vi "GetAlazar_SaveToFile - ATS-SDK.vi"(1 "File Array":string[](array[string]), 2 "lines per plane":i32, 5 "Digitizer Settings":T8={"Digitizer delay (us) "=0.0, "rf points per line"=2048, "lines per plane"=128, "Samp Rate (Hz)"=100000000.0, "Additional dig delay (us)"=0.0, "Voltage Scale"=0.4, "Pre-Looks"=0, "Offset delay (us)"=0.0, "bits A/D"=8, "Avg Num"=1, "DigTimeOut"=5.0, "Rel Dig Delay"=0.0, "Dig Ch"=0, "LeCroyCluster"={"LeCroy Channels"=[TRUE, FALSE, FALSE, FALSE], "LC read pt offset"=0.0, "Sweep Avg"=FALSE}, "Main Digitizer"=enum."NI Digitizer", "Dig Config"=enum."Single channel", "Digitizer ID Cluster"={"Acqiris/Alazar/SP ID"=[], "NI Instr Handles"=[], "LeCroy VISA"="", "GaGe Handle"={"Handle"=0, "Sample size"=0, "Resolution"=0, "Offset"=0, "Channels"=0, "Boards"=0}, "ATS Ref"="ATS9350", "Acqiris Address"=["PCI::INSTR0"], "ADQRef"=refnum, "adq_cu_ptr"=refnum}, "Trigger Settings"={"Trig Source"=1, "Trig Coupling"=0, "Trig Slope"=0, "Level (mV)"=1500.0}, "Bulk Acq"=FALSE, "Bulk Start Indexes"=[], "Data Ref RF"=refnum, "NI ID/Channel"=[], "Total Dig CH"=1, "Xtra Ann Trig delay (us)"=10.0, "Fix Z Delay?"=FALSE, "One Way Transmission?"=FALSE, "Data Ref Log"=refnum} {"Trigger Settings"."Trig Slope" items=["Positive", "Negative"]; "Trigger Settings"."Level (mV)" format="%.2f"; "Trigger Settings"."Trig Coupling" items=["DC 1 MOhm", "AC 1 MOhm", "DC 50 Ohm", "AC 50 Ohm"]; "Trigger Settings"."Trig Source" items=["Chan 1", "External"]; "Rel Dig Delay" format="%.2f"; "DigTimeOut" format="%.2f"; "Avg Num" min=1; "Offset delay (us)" format="%.2f"; "Additional dig delay (us)" format="%.2f"; "Digitizer delay (us)" format="%.2f"}, 7 "Ann Array Params":T1={"Synth Foc?"=FALSE, "Focal Zones"=41, "Switch T/R"=0, "Trans Geometry (mm)"={"Transducer"=0, "Geo Focus"=12.0, "a (radius)"=3.0, "# of rings"=5, "kerf space "=0.1, "Center Freq"=12.0}, "Sub Ap Excite?"=FALSE, "Full Array Scan?"=FALSE, "Xmt/Rcv"={"XMIT"=[TRUE, TRUE, TRUE, TRUE, TRUE], "RCV"=[TRUE, TRUE, TRUE, TRUE, TRUE]}, "PulseSpacing (us)"=0.0, "Xmit Ring"=0, "XMIT CHS"=0, "RCV CHS"=0, "GPU?"=FALSE, "Save TIFF?"=FALSE, "downfactor"=1, "RCV 1CH"=0} {"RCV 1CH" items=["All", "1", "2", "3", "4", "5"]; "Trans Geometry (mm)"."Transducer" items=["6D 12R 40 MHz"=0, "10D 31R 20 MHz"=1, "10D 23R 20 MHz"=2, "6D 23R 40 MHz"=3, "4.5D 10.7R 40 MHz"=4, "9D 23.5R 20 MHz"=5, "9D 25.8R 20MHz"=6, "Enter"=99]; "Switch T/R" min=1 max=5 step=1}, 9 "AlazarCluster":T12, 11 "errorin":errorcluster, 12 "Motion Settings":T4={"No Motion?"=FALSE, "Motion System"=enum."NI 735x", "Motion Bd ID"=1, "Motion Profile"="SMAC1", "# Axis"=1, "Reverse Z axis?"=TRUE, "SMAC Axis"=0, "scan pair"=enum."y-(x) scan", "RT fps"=6.0, "Steps per mm"=[1000, 1000, 1000, 1000], "Motor Parameters"={"velocity ct/s"=[10000.0, 10000.0, 10000.0, 50000.0], "accel ct/s^2"=[50000.0, 50000.0, 50000.0, 200000.0]}, "One Way Scan"=FALSE, "Reverse One Way Scan"=FALSE, "Global Position (mm)"=[], "Plane"=0, "Distance between\nscan lines (um)"=0.0, "Distance between\nscan planes (um)"=0.0, "number of scan planes"=1, "Total steps in line"=0, "Xtra plane\ndistance  (um)"=100, "Xtra planes "=1, "Add Axis"=FALSE, "overshoot cts"=200, "BKPT Shift"=0, "Scan Start Time (ms)"=0, "ESP VISA"="GPIB::1::INSTR", "3rd Axis"=1, "GL Ref Out"=refnum, "Galil Address"=""} {"3rd Axis" items=["x", "y", "z", "w"]; "Xtra planes" min=1; "Xtra plane\ndistance  (um)" min=0; "Distance between\nscan planes (um)" format="%.2f"; "Distance between\nscan lines (um)" format="%.2f"; "SMAC Axis" items=["None"=0, "Axis 1"=1, "Axis 2"=2, "Axis 3"=3, "Axis 4"=4, "Axis 5"=5, "Axis 6"=6, "Axis 7"=7, "Axis 8"=8, "Vector Space 1"=17, "Vector Space 2"=18, "Vector Space 3"=19, "Vector Space 4"=20]; "Motion Bd ID" min=1 max=32 step=1}, 13 "Reverse?":bool) -> (3 "Gain Array":T14(array[cluster]), 6 "VGain (dB)":dbl, 14 "Raw VGain (scale)":dbl, 15 "error out":errorcluster)   [LabVIEW 2022 SP3]
uses:
  -DigitizerRoutines/DigitizerSettings.ctl
  -DigitizerRoutines/Digitizer.ctl
  -DigitizerRoutines/DigConfig.ctl
  -DigitizerRoutines/DigitizerID.ctl
  C:/Windows/System32/ADQAPI_dotNet_helper.dll
  Motion Controllers/NI_controller/-NI_MotionRoutines/MotionParameters.ctl
  Motion Controllers/NI_controller/-NI_MotionRoutines/MotionSys.ctl
  Motion Controllers/-MotionRoutines/ScanAxis.ctl
  Motion Controllers/-MotionRoutines/3rdAxis.ctl
  Annular Array/-AnnularRoutines/AnnularArray.ctl
  Annular Array/-AnnularRoutines/TransGeometry.ctl
  Annular Array/-AnnularRoutines/ArrayGeometry.ctl
  -ScanSystem/DataHandling/ReverseData.vi
panel:
  out "Voltage Scale":T13
  # "1-D and 2-D B scan settings"
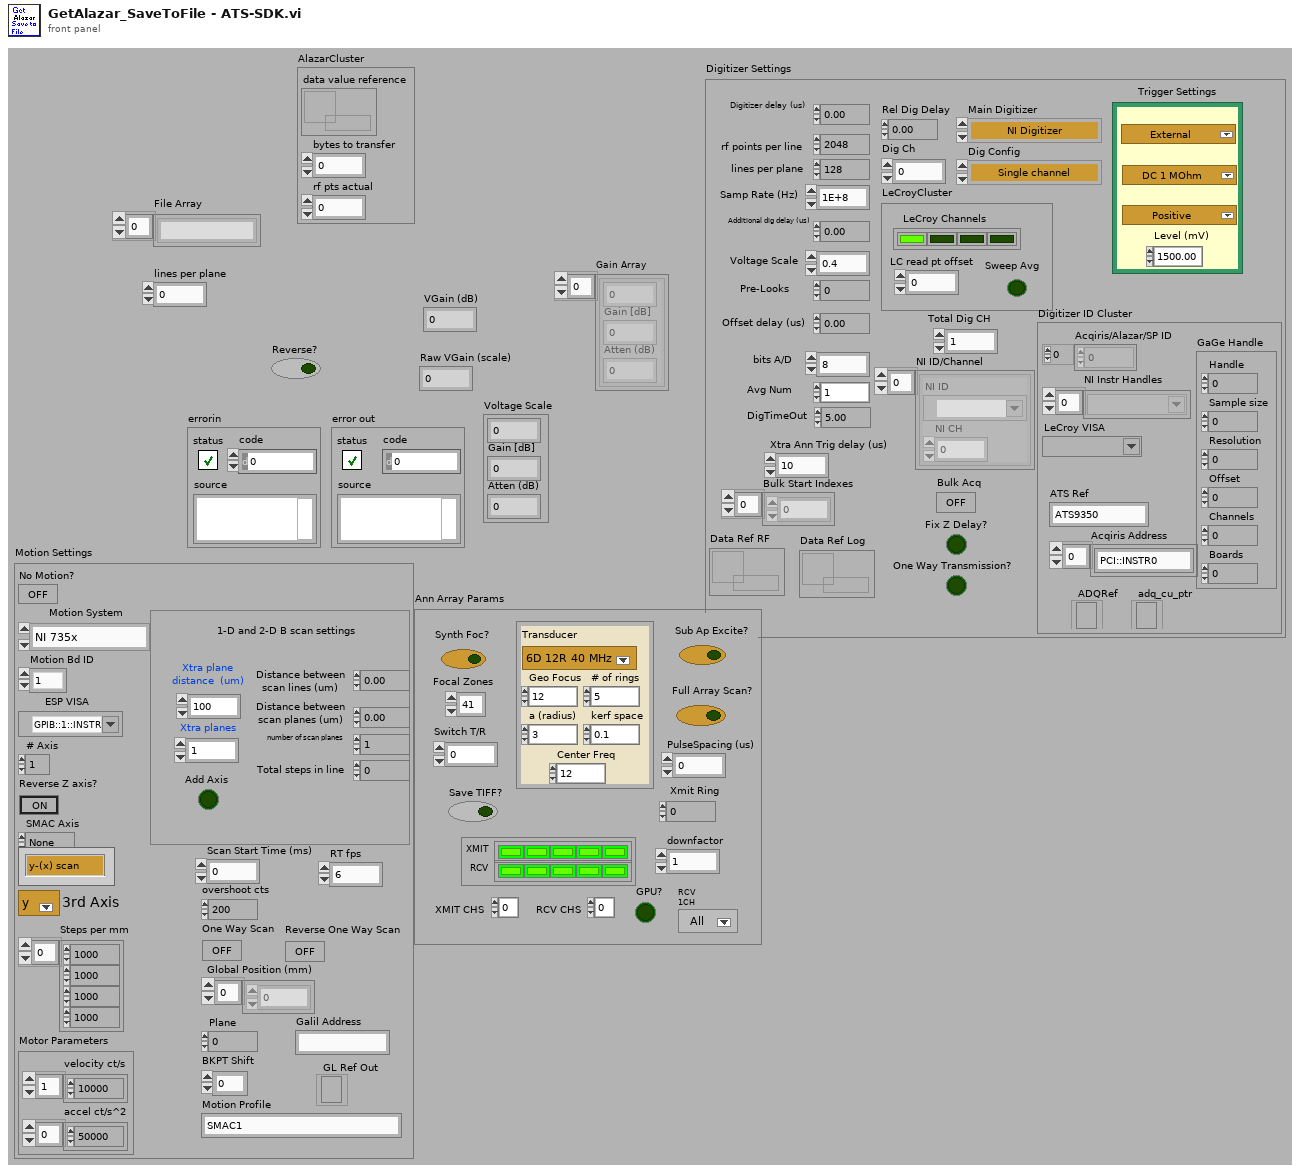
[diagram p1: front panel]
types:
  T1 = typedef "AnnularArray.ctl" = cluster{"Synth Foc?":bool, "Focal Zones":i16, "Switch T/R":i16, "Trans Geometry (mm)":T2, "Sub Ap Excite?":bool, "Full Array Scan?":bool, "Xmt/Rcv":cluster{"XMIT":bool[], "RCV":bool[]}, "PulseSpacing (us)":sgl, "Xmit Ring":i32, "XMIT CHS":u8, "RCV CHS":u8, "GPU?":bool, "Save TIFF?":bool, "downfactor":i32, "RCV 1CH":u16}
  T2 = typedef "TransGeometry.ctl" = cluster{"Transducer":T3, "Geo Focus":dbl, "a (radius)":dbl, "# of rings":i32, "kerf space ":dbl, "Center Freq":dbl}
  T3 = typedef "ArrayGeometry.ctl" = u16
  T4 = typedef "MotionParameters.ctl" = cluster{"No Motion?":bool, "Motion System":T5, "Motion Bd ID":u8, "Motion Profile":string, "# Axis":i8, "Reverse Z axis?":bool, "SMAC Axis":u16, "scan pair":T6, "RT fps":sgl, "Steps per mm":i32[], "Motor Parameters":cluster{"velocity ct/s":dbl[], "accel ct/s^2":dbl[]}, "One Way Scan":bool, "Reverse One Way Scan":bool, "Global Position (mm)":dbl[], "Plane":i32, "Distance between\nscan lines (um)":sgl, "Distance between\nscan planes (um)":sgl, "number of scan planes":i32, "Total steps in line":i32, "Xtra plane\ndistance  (um)":i32, "Xtra planes ":i32, "Add Axis":bool, "overshoot cts":i32, "BKPT Shift":i32, "Scan Start Time (ms)":u32, "ESP VISA":refnum<visa-resource-name>, "3rd Axis":T7, "GL Ref Out":refnum<k7>, "Galil Address":string}
  T5 = typedef "MotionSys.ctl" = enum16{"MM3000", "NI 735x", "Newport ESP", "No Motion Card", "Galil"}
  T6 = typedef "ScanAxis.ctl" = enum16{"y-(x) scan", "x-(y) scan", "z-(x) scan", "z-(y) scan", "y-(z) scan", "x-(z) scan", "w-(x) scan", "w-(y) scan", "w-(z) scan", "x-(w) scan", "y-(w) scan", "z-(w) scan"}
  T7 = typedef "3rdAxis.ctl" = u16
  T8 = typedef "DigitizerSettings.ctl" = cluster{"Digitizer delay (us) ":dbl, "rf points per line":i32, "lines per plane":i32, "Samp Rate (Hz)":dbl, "Additional dig delay (us)":dbl, "Voltage Scale":dbl, "Pre-Looks":i32, "Offset delay (us)":dbl, "bits A/D":i8, "Avg Num":i32, "DigTimeOut":sgl, "Rel Dig Delay":sgl, "Dig Ch":i32, "LeCroyCluster":cluster{"LeCroy Channels":bool[], "LC read pt offset":dbl, "Sweep Avg":bool}, "Main Digitizer":T9, "Dig Config":T10, "Digitizer ID Cluster":T11, "Trigger Settings":cluster{"Trig Source":u16, "Trig Coupling":u16, "Trig Slope":u16, "Level (mV)":dbl}, "Bulk Acq":bool, "Bulk Start Indexes":i32[], "Data Ref RF":refnum<data-value>, "NI ID/Channel":cluster{"NI ID":refnum<k15>, "NI CH":i32}[], "Total Dig CH":i32, "Xtra Ann Trig delay (us)":dbl, "Fix Z Delay?":bool, "One Way Transmission?":bool, "Data Ref Log":refnum<data-value>}
  T9 = typedef "Digitizer.ctl" = enum16{"Acqiris Digitizer", "NI Digitizer", "LeCroy", "GaGe", "AlazarTech", "No Digitizer", "Teledyne"}
  T10 = typedef "DigConfig.ctl" = enum16{"Single channel", "2 Chans w/ 2 Acqiris", "2 Chans w/ 1 Acqiris", "5-CH Pulser New", "5-CH pulser w/ ann array", "5-pass style ann array", "Empty"}
  T11 = typedef "DigitizerID.ctl" = cluster{"Acqiris/Alazar/SP ID":u32[], "NI Instr Handles":refnum<k15>[], "LeCroy VISA":refnum<visa-resource-name>, "GaGe Handle":cluster{"Handle":u32, "Sample size":u32, "Resolution":i32, "Offset":i32, "Channels":u32, "Boards":u32}, "ATS Ref":string, "Acqiris Address":string[], "ADQRef":refnum<k24>, "adq_cu_ptr":refnum<k24>}
  T12 = cluster{"data value reference":refnum<data-value>, "bytes to transfer":u32, "rf pts actual":u32}
  T13 = cluster{sgl, "Gain [dB]  ":sgl, "Atten (dB)":sgl}
  T14 = cluster{sgl, "Gain [dB]  ":sgl, "Atten (dB)":sgl}[]
  T15 = enum16{"big-endian, network order", "native, host order", "little-endian"}
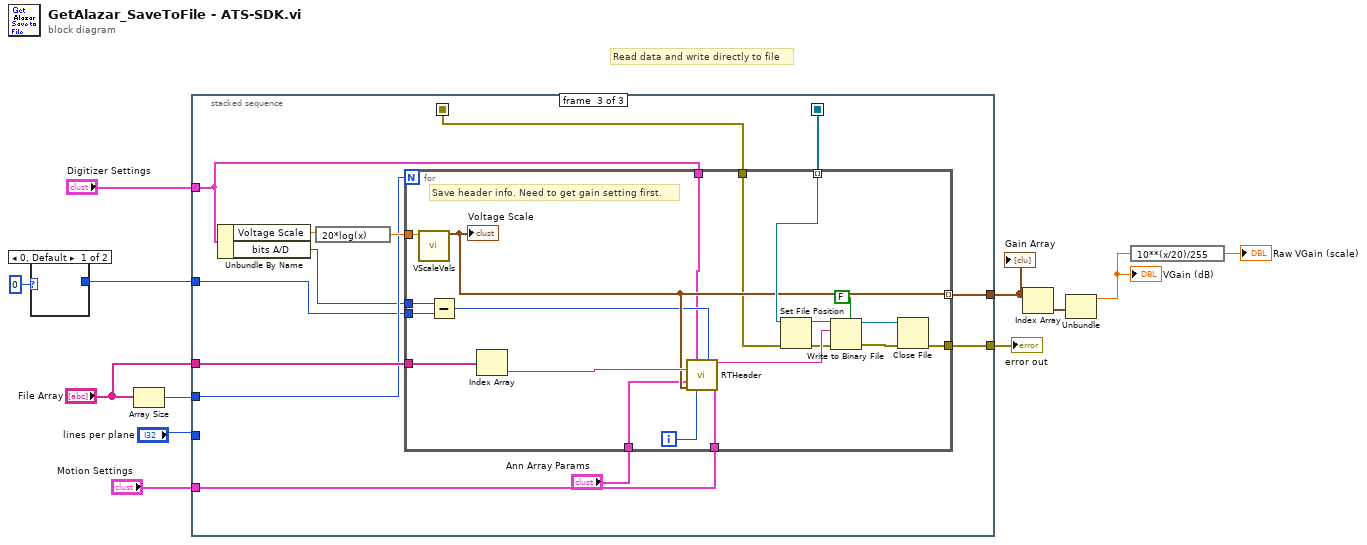
[diagram p0: block diagram]
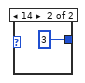
[diagram p2: hidden frame]
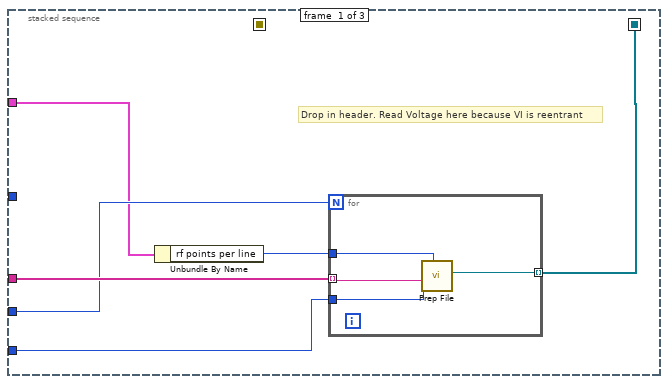
[diagram p3: hidden frame]
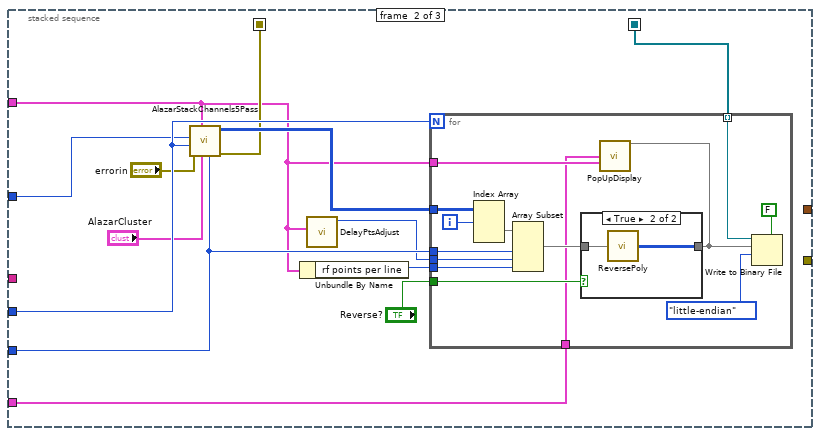
[diagram p4: hidden frame]
diagram:
  # "Read data and write directly to file"
  n1 = case shown="0, Default" i8 0 ("bits A/D") {
    tunnel: [_ u16 3 ("Extra Shift")] -> w5
    frame 0, Default {
    }
    frame 14 {
    }
  }
  n2 = Array Size(array="File Array") -> (size(s)=w9:i32)
  n3 = stacked-sequence {
    seq-local: [w19 _ _] -> [_ w34 w61]
    seq-local: [_ w29 _] -> [_ _ w57]
    tunnel: [_ _ w66] -> w2
    tunnel: "lines per plane" -> [w17 w35 _]
    tunnel: "File Array" -> [w18 _ w65]
    tunnel: w9 -> [w16 w33 w62]
    tunnel: [_ _ w63] -> w6
    tunnel: w5 -> [_ w31 w60]
    tunnel: "Digitizer Settings" -> [w15 w25 w56]
    tunnel: "Motion Settings" -> [_ w32 w58]
    frame #0 {
      # "Drop in header. Read Voltage here because VI is reentrant"
      n4 = Unbundle By Name(w15) -> ("rf points per line"=w14:i32)
      n5 = for {
        N: w16 -> [_]
        tunnel: [w23] -> w19 mode=indexing
        tunnel: w18 -> [w20] mode=indexing
        tunnel: w14 -> [w22]
        tunnel: w17 -> [w21]
        n6 = call "Prep File.vi"("Num Samps"=w22, "Num Segs"=w21, "File Name"=w20) -> ("refnum out"=w23:refnum<file>)  [unwired: 4 in, 1 out]
      }
    }
    frame #1 {
      n7 = call "AlazarStackChannels5Pass.vi"("lines per plane"=w35, "AlazarCluster"="AlazarCluster", "Digitizer Settings"=w25, "error in"="errorin", "Channels"=w33, "Extra Shift"=w31) -> ("error out"=w29:errorcluster, "ChStackDataOut"=w36:i16[][][])  [unwired: 2 in, 2 out]
      n8 = Unbundle By Name(w25) -> ("rf points per line"=w28:i32)
      n9 = call "DelayPtsAdjust.vi"("Digitizer Settings"=w25) -> ("PostDelayCorrection"=w24:u32)  [unwired: 9 in, 1 out]
      n10 = for {
        N: w33 -> [_]
        tunnel: w36 -> [w50]
        tunnel: w28 -> [w49]
        tunnel: w35 -> [w48]
        tunnel: "Reverse?" -> [w47]
        tunnel: w34 -> [w43] mode=indexing
        tunnel: w25 -> [w39]
        tunnel: w32 -> [w38]
        tunnel: w24 -> [w37]
        i -> [w41]
        n11 = Index Array(array=w50, index (dim 0)=w41) -> (element=w42:i16[][])  [unwired: 2 in]
        n12 = Array Subset(array=w42, length (row)=w48, index (col)=w37, length (col)=w49) -> (w46:i16[][])  [unwired: 1 in]
        n13 = case shown="True" w47 {
          tunnel: [w51 w53] -> w40
          tunnel: w46 -> [w51 w52]
          frame False {
          }
          frame True {
            n14 = call-poly "ReversePoly.vi"("Array in"=w52) -> ("Array out"=w53:i16[][])
          }
        }
        n15 = call "PopUpDisplay.vi"("Data"=w40, "Motion Settings In"=w38, "Digitizer Settings"=w39) -> ()  [unwired: 13 in]
        n16 = Write to Binary File(file (use dialog)=w43, data=w40, 5:FALSE ("prepend array or string size? (T)"), 9:T15."little-endian" ("byte order (0:big-endian, network order)")) -> ()  [unwired: 2 in, 3 out]
      }
    }
    frame #2 {
      n17 = Unbundle By Name(w56) -> ("Voltage Scale"=w55:dbl, "bits A/D"=w54:i8)
      n18 = expression code="20*log(x)"(w55) -> (w64:dbl)
      n19 = for {
        N: w62 -> [_]
        tunnel: [w86] -> w66
        tunnel: w65 -> [w85]
        tunnel: [w75] -> w63 mode=indexing
        tunnel: w64 -> [w77]
        tunnel: w61 -> [w76] mode=indexing
        tunnel: w60 -> [w74]
        tunnel: w56 -> [w72]
        tunnel: w58 -> [w71]
        tunnel: "Ann Array Params" -> [w69]
        tunnel: w57 -> [w68]
        tunnel: w54 -> [w67]
        i -> [w70]
        # "Save header info. Need to get gain setting first."
        n20 = call "VScaleVals.vi"("Full Scale"=w77) -> ("Voltage Scale"=w75:T13)  [unwired: 8 in, 2 out]
        "Voltage Scale" <- w75
        n21 = Subtract(x=w67, y=w74) -> (x-y=w73:u16)
        n22 = Index Array(array=w85) -> (element=w78:string)  [unwired: 1 in]
        n23 = call "RTHeader.vi"("Digitizer Settings"=w72, "Dig Word Size"=w73, "File Name In"=w78, "Ann Array Params"=w69, "Votage scaling"=w75, "Pulser Channel"=w70, "Motion Settings"=w71) -> ("Header String Out"=w81:string)  [unwired: 7 in, 1 out]
        n24 = Set File Position(refnum=w76, error in=w68) -> (refnum out=w80:refnum<file>, error out=w79:errorcluster)  [unwired: 2 in]
        n25 = Write to Binary File(file (use dialog)=w80, data=w81, error in=w79, 5:FALSE ("prepend array or string size? (T)")) -> (refnum out=w83:refnum<file>, error out=w82:errorcluster)  [unwired: 2 in, 1 out]
        n26 = Close File(refnum=w83, error in=w82) -> (error out=w86:errorcluster)  [unwired: 1 out]
      }
    }
  }
  "Gain Array" <- w6
  "error out" <- w2
  n27 = Index Array(array=w6) -> (element=w10:T13)  [unwired: 1 in]
  n28 = Unbundle(w10) -> (w11:sgl)  [unwired: 2 out]
  "VGain (dB)" <- w11
  n29 = expression code="10**(x/20)/255"(w11) -> (→"Raw VGain (scale)":sgl)
